vi "Spectrum over time.vi"() -> ()   [LabVIEW 2021]
uses:
  <vilib>/Utility/error.llb/DialogType.ctl
  cb6d7afe-07a1-4717-8708-8a88368bf63c.vi
panel:
  in  "Ref Level Auto":bool=TRUE
  out "Min":dbl
  out "Sec":dbl
  out "H":dbl
  in  "Stop Button":bool
  out "P x Lambda Graph":cluster{dbl[], dbl[]}(graph)
  out "Corrente Atual (mA)":dbl
  out "P x I Graph":cluster{dbl[], dbl[]}(graph)
  in  "Start Button":bool
  in  "Cluster de Dados de Entrada":T1={"Corrente Inicial (mA)"=30.0, "Limite de Temperatura"=27.0, "Temperatura"=25.0, "Corrente Limite (mA)"=300, "Centralizar pico (nm)"=1557.0, "Valor de Span (nm)"=20.0, "Passo (mA)"=10.0, "Corrente Final (mA)"=650.0, "Resolucao"=enum."High", "Modo"=enum."Laser"} {"Corrente Final (mA)" min=0.0 step=1.0; "Passo (mA)" min=1.0 step=1.0; "Valor de Span (nm)" min=0.1 max=1400.0 format="%.2f"; "Centralizar pico (nm)" format="%.2f"; "Temperatura" min=-100.0 max=199.9 step=0.1; "Limite de Temperatura" min=-100.0 max=199.9 step=0.1; "Corrente Inicial (mA)" min=0.0 step=1.0}
  out "XY Graph":T2(graph)
  in  "Pasta Destino":path=path "d:/Users/acquisition"
  in  "GPIB Analisador de Espectros":refnum<visa-resource-name>="Advantest_Spectrometer_82357A"
  in  "GPIB Controlador Laser Diodo":refnum<visa-resource-name>="DiodeLaserController__82357A"
  in  "error in (no error)":errorcluster
  out "error out":errorcluster
  # "Tempo Gasto"
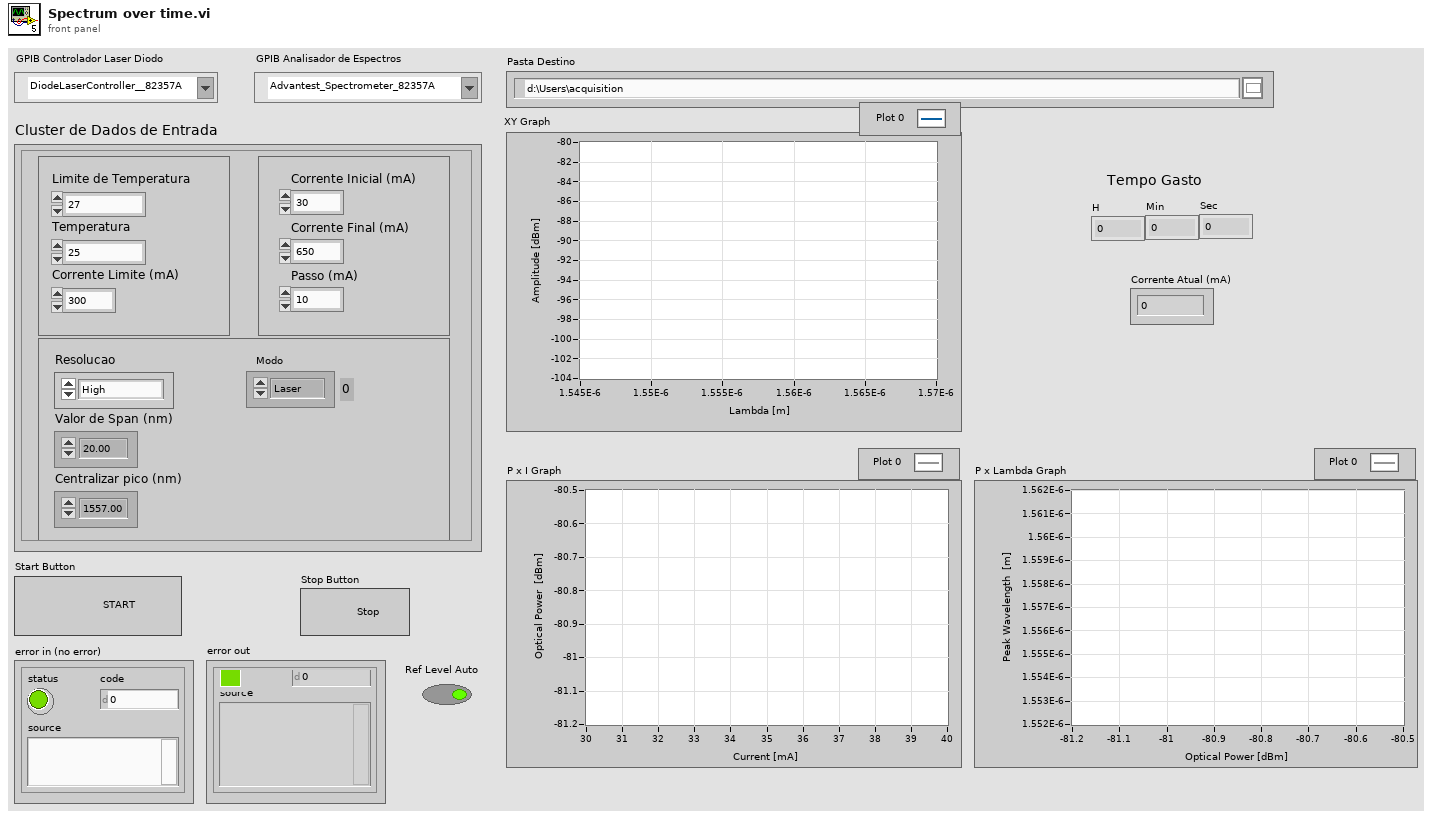
[diagram p1: front panel]
types:
  T1 = cluster{"Corrente Inicial (mA)":dbl, "Limite de Temperatura":dbl, "Temperatura":dbl, "Corrente Limite (mA)":i32, "Centralizar pico (nm)":dbl, "Valor de Span (nm)":dbl, "Passo (mA)":dbl, "Corrente Final (mA)":dbl, "Resolucao":enum16{"Normal", "High"}, "Modo":enum16{"Laser", "Led"}}
  T2 = cluster{"Wavelike Data":dbl[], "Wavelike Data":dbl[]}
  T3 = typedef "DialogType.ctl" = u16
  T4 = cluster{"Limite de Temperatura":dbl, "Temperatura":dbl, "Corrente Inicial (mA)":dbl, "Corrente Limite (mA)":i32, "Resolucao":enum16{"Normal", "High"}, "Centralizar pico (nm)":dbl, "Valor de Span (nm)":dbl, "Modo":enum16{"Laser", "Led"}}
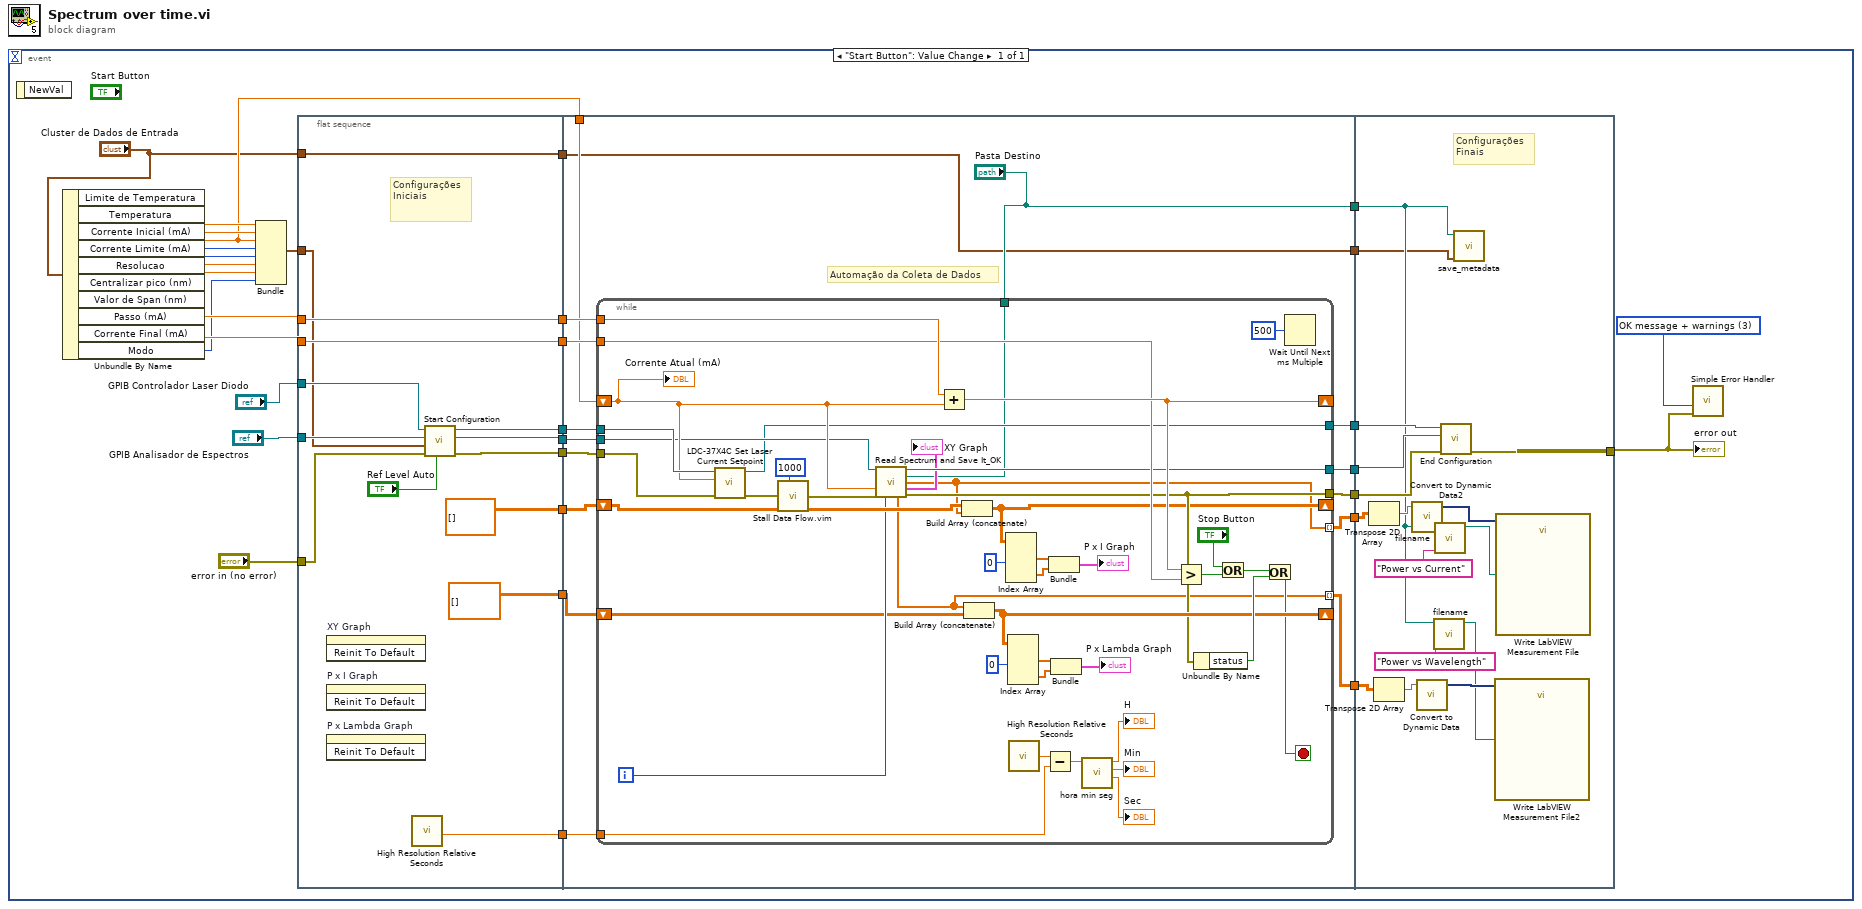
[diagram p0: block diagram]
diagram:
  n1 = event shown="[0] \"Start Button\": Value Change" {
    selector: _ -> [_]
    dyn-events: _ -> [_]
    timeout: _ -> [_]
    event "Start Button": Value Change {
      w10 = T3 3 items=["no dialog", "OK message", "continue or stop message", "OK message + warnings", "continue/stop + warnings"] ("type of dialog (OK msg:1)")
      n2 = event-data() -> ()  [unwired: 1 in, 1 out]
      n3 = Unbundle By Name("Cluster de Dados de Entrada") -> ("Limite de Temperatura"=w24:dbl, "Temperatura"=w23:dbl, "Corrente Inicial (mA)"=w15:dbl, "Corrente Limite (mA)"=w22:i32, "Resolucao"=w21:enum16{"Normal", "High"}, "Centralizar pico (nm)"=w20:dbl, "Valor de Span (nm)"=w18:dbl, "Passo (mA)"=w17:dbl, "Corrente Final (mA)"=w16:dbl, "Modo"=w1:enum16{"Laser", "Led"})
      n4 = Bundle("Limite de Temperatura"=w24, "Temperatura"=w23, "Corrente Inicial (mA)"=w15, "Corrente Limite (mA)"=w22, "Resolucao"=w21, "Centralizar pico (nm)"=w20, "Valor de Span (nm)"=w18, "Modo"=w1) -> (w19:T4)  [unwired: 1 in]
      n5 = flat-sequence {
        tunnel: "error in (no error)" -> [w39]
        tunnel: [w47] -> w33
        tunnel: [w46] -> w32
        tunnel: "GPIB Controlador Laser Diodo" -> [w45]
        tunnel: "GPIB Analisador de Espectros" -> [w44]
        tunnel: [w43] -> w31
        tunnel: [w42] -> w30
        tunnel: w17 -> [w42]
        tunnel: w16 -> [w41]
        tunnel: [w41] -> w29
        tunnel: w19 -> [w34]
        tunnel: [dbl[][] []] -> w14
        tunnel: [dbl[][] []] -> w9
        tunnel: [w37] -> w8
        tunnel: [w36] -> w4
        tunnel: "Cluster de Dados de Entrada" -> [w36]
        tunnel: w33 -> [w63]
        tunnel: w32 -> [w62]
        tunnel: w31 -> [w61]
        tunnel: [w60] -> w28
        tunnel: w30 -> [w59]
        tunnel: w29 -> [w58]
        tunnel: w15 -> [w57]
        tunnel: w14 -> [w56]
        tunnel: [w55] -> w13
        tunnel: [w54] -> w12
        tunnel: w9 -> [w53]
        tunnel: w8 -> [w52]
        tunnel: ["Pasta Destino"] -> w7
        tunnel: [w50] -> w6
        tunnel: [w49] -> w5
        tunnel: w4 -> [w48]
        tunnel: [w48] -> w3
        tunnel: [w121] -> w11
        tunnel: w28 -> [w120]
        tunnel: w13 -> [w119]
        tunnel: w12 -> [w118]
        tunnel: w7 -> [w107]
        tunnel: w6 -> [w109]
        tunnel: w5 -> [w111]
        tunnel: w3 -> [w106]
        frame #0 {
          # "Configurações\nIniciais"
          n6 = invoke on="XY Graph" class="XYGraph (strict)" method="Reinit To Default"() -> ()  [unwired: 3 in, 3 out]
          n7 = invoke on="P x I Graph" class="XYGraph (strict)" method="Reinit To Default"() -> ()  [unwired: 3 in, 3 out]
          n8 = invoke on="P x Lambda Graph" class="XYGraph (strict)" method="Reinit To Default"() -> ()  [unwired: 3 in, 3 out]
          n9 = call <vilib>:"High Resolution Relative Seconds.vi"() -> ("relative seconds"=w37:dbl)
          n10 = call "Start Configuration.vi"("Ref Lvl Auto"="Ref Level Auto", "error in (no error)"=w39, "Cluster de Dados"=w34, "GPIB Espectrometro"=w44, "GPIB Controlador Laser Diodo"=w45) -> ("error out"=w47:errorcluster, "Spectrometer out"=w43:refnum<visa-resource-name>, "Controller out"=w46:refnum<visa-resource-name>)  [unwired: 4 in]
        }
        frame #1 {
          # "Automação da Coleta de Dados"
          n11 = while {
            shift-right: [w99] -> _
            shift-left: w57 -> [w100]
            tunnel: w63 -> [w92]
            tunnel: w62 -> [w105]
            tunnel: w61 -> [w98]
            tunnel: [w95] -> w60
            tunnel: w59 -> [w97]
            tunnel: w58 -> [w96]
            shift-right: [w66] -> _
            shift-left: w56 -> [w91]
            tunnel: [w79] -> w55
            tunnel: [w86] -> w54
            shift-right: [w80] -> _
            shift-left: w53 -> [w81]
            tunnel: w52 -> [w75]
            tunnel: "Pasta Destino" -> [w67]
            tunnel: [w65] -> w50 mode=indexing
            tunnel: [w64] -> w49 mode=indexing
            i -> [w87]
            stop <- w77 stop-if-true
            n12 = call "LDC-37X4C Set Laser Current Setpoint.vi"("error in (no error)"=w92, "Current"=w100, "VISA resource name"=w105) -> ("error out"=w103:errorcluster, "VISA resource name out"=w95:refnum<visa-resource-name>)  [unwired: 7 in]
            n13 = call "Stall Data Flow.vim"("value in"=w103, "milliseconds to wait"=u32 1000) -> ("value out"=w101:errorcluster)  [unwired: 1 out]
            n14 = call "Read Spectrum and Save It_OK.vi"("VISA Session"=w98, "Pasta Destino DESTA aquisicao"=w67, "Corrente Atual (mA)"=w100, "Error In"=w101, "Iteracao"=w87) -> ("Copy VISA Session"=w86:refnum<visa-resource-name>, "PxI"=w64:dbl[], "XY Graph"=→"XY Graph":T2, "PxLambda"=w65:dbl[], "Error Out"=w79:errorcluster)  [unwired: 4 in, 2 out]
            n15 = Add(x=w97, y=w100) -> (x+y=w99:dbl)
            n16 = Build Array (concatenate)(w91, w64) -> (w66:dbl[][])
            n17 = Build Array (concatenate)(w65, w81) -> (w80:dbl[][])
            n18 = Index Array(array=w66, index (col) #1=0 ("disabled index (col)")) -> (element #1=w89:dbl[], element #2=w88:dbl[])  [unwired: 3 in]
            n19 = Index Array(array=w80, index (col) #1=0 ("disabled index (col)")) -> (element #1=w83:dbl[], element #2=w82:dbl[])  [unwired: 3 in]
            n20 = call <vilib>:"High Resolution Relative Seconds.vi"() -> ("relative seconds"=w76:dbl)
            n21 = Subtract(x=w76, y=w75) -> (x-y=w74:dbl)
            n22 = Bundle(w89, w88) -> (→"P x I Graph":cluster{dbl[], dbl[]})  [unwired: 1 in]
            n23 = Bundle(w83, w82) -> (→"P x Lambda Graph":cluster{dbl[], dbl[]})  [unwired: 1 in]
            n24 = call "hora min seg.vi"("Total time in seconds"=w74) -> ("Sec"=→"Sec":dbl, "Min"=→"Min":dbl, "H"=→"H":dbl)  [unwired: 8 in]
            n25 = Greater?(x=w99, y=w96) -> (0:w102:bool)
            n26 = Unbundle By Name(w79) -> ("status"=w93:bool)
            n27 = Or(x="Stop Button", y=w102) -> (x .or. y?=w94:bool)
            n28 = Or(x=w94, y=w93) -> (x .or. y?=w77:bool)
            n29 = Wait Until Next ms Multiple(millisecond multiple=u32 500) -> ()  [unwired: 1 out]
            "Corrente Atual (mA)" <- w100
          }
        }
        frame #2 {
          # "Configurações\nFinais"
          n30 = Transpose 2D Array(2D array=w111) -> (transposed array=w110:dbl[][])
          n31 = Transpose 2D Array(2D array=w109) -> (transposed array=w108:dbl[][])
          n32 = call "Convert to Dynamic Data2"("2D Array"=w110) -> ("Dynamic Data Type"=w114:dynamicdata)  [unwired: 3 in]
          n33 = call "Convert to Dynamic Data"("2D Array"=w108) -> ("Dynamic Data Type"=w115:dynamicdata)  [unwired: 3 in]
          n34 = call "filename.vi"("Filename"="Power vs Wavelength", "Pasta Destino"=w107) -> ("filename output"=w112:path)  [unwired: 9 in]
          n35 = call "filename.vi"("Filename"="Power vs Current", "Pasta Destino"=w107) -> ("filename output"=w113:path)  [unwired: 9 in]
          n36 = call "End Configuration.vi"("error in (no error)"=w119, "GPIB Espectrometro"=w118, "GPIB Controlador Laser Diodo"=w120) -> ("error out"=w121:errorcluster)  [unwired: 8 in]
          n37 = call "save_metadata.vi"("Cluster de Dados de Entrada"=w106, "Pasta Destino"=w107) -> ()  [unwired: 10 in]
          n38 = call "Write LabVIEW Measurement File2"("Signals"=w115, "Filename"=w112) -> ()  [unwired: 15 in, 3 out]
          n39 = call "Write LabVIEW Measurement File"("Signals"=w114, "Filename"=w113) -> ()  [unwired: 15 in, 3 out]
        }
      }
      n40 = call <vilib>:"Simple Error Handler.vi"("type of dialog (OK msg:1)"=w10, "error in (no error)"=w11) -> ()  [unwired: 3 in, 5 out]
      "error out" <- w11
    }
  }
